vi "_RT Event.vi"(4 "error in (no error)":errorcluster, 5 "Event":string, 7 "Action (Write)":enum16{"Write", "Read"}(ring)) -> (0 "error out":errorcluster, 1 "Log":string)   [LabVIEW 2012]
uses:
  _RT Global.vi
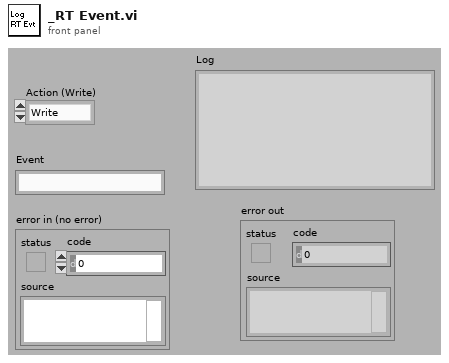
[diagram p1: front panel]
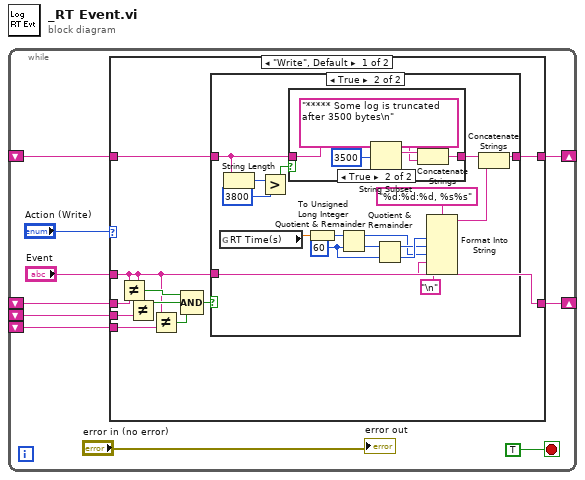
[diagram p0: block diagram]
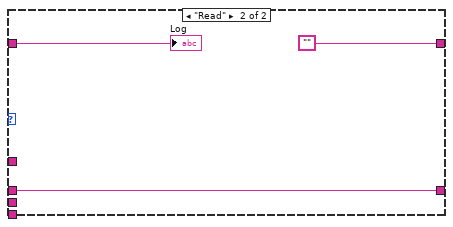
[diagram p4: hidden frame]
diagram:
  n1 = while {
    shift-right: [w9] -> _
    shift-left: _ -> [w8]
    shift-right: [w4] -> _
    shift-left: _ -> [w3]
    shift-left: _ -> [w2]
    shift-left: _ -> [w1]
    stop <- TRUE stop-if-true
    n2 = case shown="\"Write\", Default" "Action (Write)" {
      tunnel: [w19 ""] -> w9
      tunnel: w8 -> [w20 w47]
      tunnel: "Event" -> [w12 _]
      tunnel: [w12 w45] -> w4
      tunnel: w3 -> [w18 w45]
      tunnel: w2 -> [w17 _]
      tunnel: w1 -> [w13 _]
      frame "Write", Default {
        n3 = Not Equal?(x=w12, y=w18) -> (x != y?=w15:bool)
        n4 = Not Equal?(x=w12, y=w17) -> (x != y?=w14:bool)
        n5 = Not Equal?(x=w12, y=w13) -> (x != y?=w11:bool)
        n6 = Compound Arithmetic op=AND(w15, w14, w11) -> (w16:bool)
        n7 = case shown="True" w16 {
          tunnel: w20 -> [w21 w23]
          tunnel: [w21 w29] -> w19
          tunnel: w12 -> [_ w27]
          frame False {
          }
          frame True {
            w38 = u32 60 ("y")
            n8 = global read "_RT Global.vi" "RT Time(s)"() -> (w35:dbl)
            n9 = String Length(string=w23) -> (length=w26:i32)
            n10 = Greater?(x=w26, y=3800) -> (0:w24:bool)
            n11 = case shown="True" w24 {
              tunnel: w23 -> [w39 w44]
              tunnel: [w39 w42] -> w22
              frame False {
              }
              frame True {
                n12 = String Subset(string=w44, offset (0)=3500) -> (substring=w41:string)  [unwired: 1 out]
                n13 = Concatenate Strings(w41, "***** Some log is truncated after 3500 bytes\n") -> (w42:string)
              }
            }
            n14 = To Unsigned Long Integer(number=w35) -> (unsigned 32bit integer=w36:u32)
            n15 = Quotient & Remainder(x=w36, y=w38) -> (x-y*floor(x/y)=w32:u32, floor(x/y)=w37:u32)
            n16 = Quotient & Remainder(x=w37, y=w38) -> (x-y*floor(x/y)=w33:u32, floor(x/y)=w34:u32)
            n17 = Format Into String(format string="%d:%d:%d, %s%s", w34, w33, w32, w27, "\n") -> (resulting string=w30:string)  [unwired: 2 in, 1 out]
            n18 = Concatenate Strings(w22, w30) -> (w29:string)
          }
        }
      }
      frame "Read" {
        "Log" <- w47
      }
    }
    "error out" <- "error in (no error)"
  }
